vi "EvaluateTimers.vi"(8 "error in (no error)":errorcluster, 11 "timer in":T1[](array[typedef])) -> (0 "error out":errorcluster, 3 "timer out":T1[](array[typedef]))   [LabVIEW 2017, in "TimerProcess.lvlib"]
uses:
  <vilib>/addons/TimerProcess/TimerProcess.lvlib
  <vilib>/addons/TimerProcess/controls/internalTask.ctl
  <vilib>/addons/Qbus/Qbus.lvclass
  <vilib>/addons/TimerProcess/controls/taskType.ctl
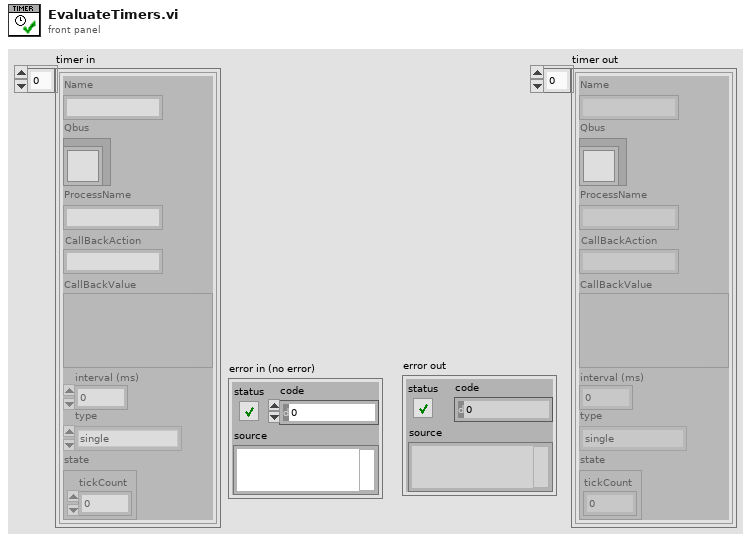
[diagram p1: front panel]
types:
  T1 = typedef "TimerProcess.lvlib/internalTask.ctl" = cluster{"Name":string, "Qbus":refnum<class "Qbus.lvclass">, "ProcessName":string, "CallBackAction":string, "CallBackValue":variant, "interval (ms)":i32, "type":T2, "state":cluster{"tickCount":u32}}
  T2 = typedef "TimerProcess.lvlib/taskType.ctl" = enum16{"single", "repeat"}
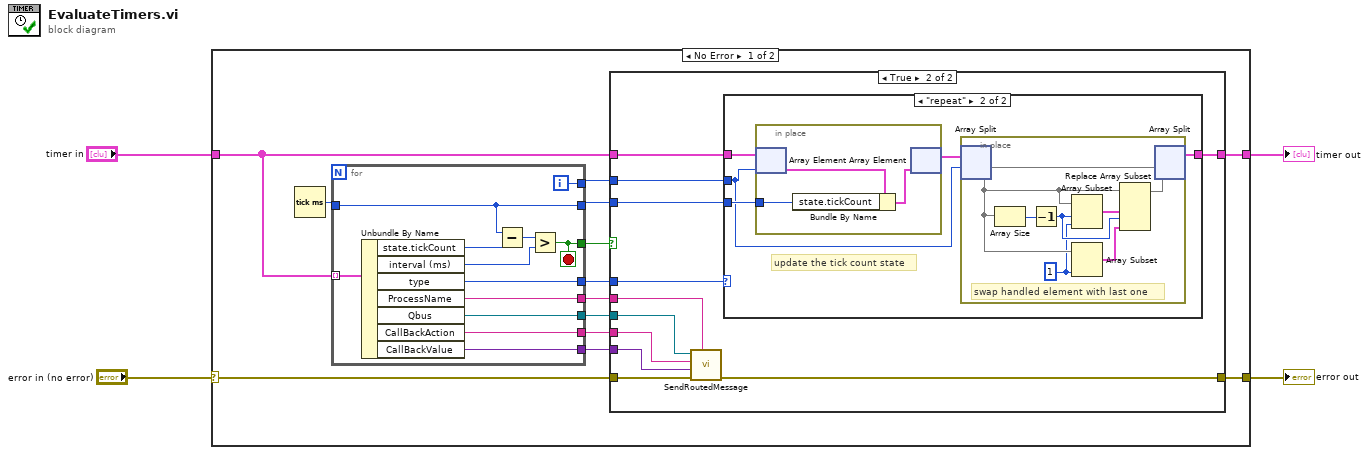
[diagram p0: block diagram]
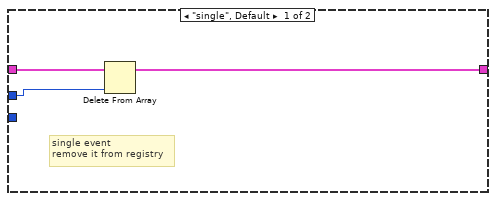
[diagram p3: hidden frame]
diagram:
  n1 = case shown="No Error" "error in (no error)" {
    selector: "error in (no error)" -> [w6 w63]
    tunnel: "timer in" -> [w17 w62]
    tunnel: [w16 w62] -> w3
    tunnel: [w15 w63] -> w2
    frame No Error {
      n2 = Tick Count (ms)() -> (millisecond timer value=w14:u32)
      n3 = for {
        tunnel: w17 -> [w60] mode=indexing
        tunnel: [w54] -> w11
        tunnel: [w58] -> w10
        tunnel: [w56] -> w12
        tunnel: [w57] -> w13
        tunnel: w14 -> [w56]
        tunnel: [w55] -> w9
        tunnel: [w53] -> w8
        tunnel: [w51] -> w7
        tunnel: [w50] -> w5
        i -> [w57]
        stop <- w58 stop-if-true
        n4 = Unbundle By Name(w60) -> ("state.tickCount"=w52:u32, "interval (ms)"=w59:i32, "type"=w53:T2, "ProcessName"=w54:string, "Qbus"=w50:refnum<class "Qbus.lvclass">, "CallBackAction"=w55:string, "CallBackValue"=w51:variant)
        n5 = Subtract(x=w56, y=w52) -> (x-y=w61:u32)
        n6 = Greater?(x=w61, y=w59) -> (0:w58:bool)
      }
      n7 = case shown="True" w10 {
        tunnel: w11 -> [_ w21]
        tunnel: w12 -> [_ w26]
        tunnel: w13 -> [_ w28]
        tunnel: w6 -> [w19 w24]
        tunnel: [w19 w25] -> w15
        tunnel: w9 -> [_ w23]
        tunnel: w8 -> [_ w30]
        tunnel: [w18 w29] -> w16
        tunnel: w17 -> [w18 w27]
        tunnel: w7 -> [_ w22]
        tunnel: w5 -> [_ w20]
        frame False {
        }
        frame True {
          n8 = call <vilib>:"SendRoutedMessage.vi"("listener process"=w21, "error in (no error)"=w24, "message value"=w22, "message name"=w23, "Qbus in"=w20) -> ("error in (no error)"=w25:errorcluster)  [unwired: 5 in, 1 out]
          n9 = case shown="\"repeat\"" w30 {
            tunnel: [w33 w34] -> w29
            tunnel: w28 -> [w32 w35]
            tunnel: w27 -> [w31 w38]
            tunnel: w26 -> [_ w37]
            frame "single", Default {
              # "single event\nremove it from registry"
              n10 = Delete From Array(array=w31, index=w32) -> (array with subset deleted=w33:T1[])  [unwired: 1 in, 1 out]
            }
            frame "repeat" {
              # "update the tick count state"
              n11 = in-place {
                in-place-border: w37 -> [w48]
                n12 = in-place-array #1(w38, w35) -> (w49:T1)
                n13 = Bundle By Name(cluster=w49, "state.tickCount"=w48) -> (w47:T1)
                n14 = in-place-array #1(w47) -> (w36:T1[])  [unwired: 1 out]
              }
              n15 = in-place {
                w39 = 1 ("length")
                # "swap handled element with last one"
                n16 = in-place-split #2(w36, w35) -> (w46:T1[], w45:T1[])
                n17 = Array Size(array=w45) -> (size(s)=w42:i32)
                n18 = Decrement(x=w42) -> (x-1=w40:i32)
                n19 = Array Subset(array=w45, index=w40, length=w39) -> (w44:T1[])
                n20 = Array Subset(array=w45, length=w39) -> (w43:T1[])  [unwired: 1 in]
                n21 = Replace Array Subset(array=w45, new element #1=w44, new element #2=w43, index #2=w40) -> (w41:T1[])  [unwired: 1 in]
                n22 = in-place-split #2(w46, w41) -> (w34:T1[])  [unwired: 1 out]
              }
            }
          }
        }
      }
    }
    frame Error {
    }
  }
  "timer out" <- w3
  "error out" <- w2
